vi "SL TAGS Open.vi"(8 "error in (no error)":errorcluster, 10 "Tag Properties":T1[](array[typedef]), 11 "EEISysLink in":refnum<class "EEISysLink.lvclass">) -> (0 "error out":errorcluster, 3 "EEISysLink out":refnum<class "EEISysLink.lvclass">)   [LabVIEW 2017, in "EEISysLink.lvclass"]
doc: "Open a local instance for each tag in a list per the input properties. Opened tags will be placed in the class data.\n\nThis does not synchronize them with a SystemLink server. To do that call the \"Ceate-Sync Server method\".\n\nJames Tillett\nEndeavor Engineering Inc.\nwww.endeavoreng.com"
uses:
  EEISysLink.lvclass
  Controls/SL Tag Properties.ctl
  Controls/SL Tag Data Type.ctl
  Controls/SL Tag Interpolation Method.ctl
  Controls/SL Tag Unit of Measure.ctl
  Controls/SL Tag Type.ctl
  <vilib>/Skyline/Configuration/Configuration_class/NI Skyline Configuration.lvclass
  <vilib>/Skyline/Configuration/Configuration AMQP_class/NI Skyline Configuration AMQP.lvclass
  C:/Program Files (x86)/National Instruments/LabVIEW 2017/vi.lib/Skyline/Configuration/Configuration_class/NI Skyline Configuration.lvclass
  <vilib>/Skyline/Configuration/Configuration AMQP_class/Open Configuration AMQP.vi
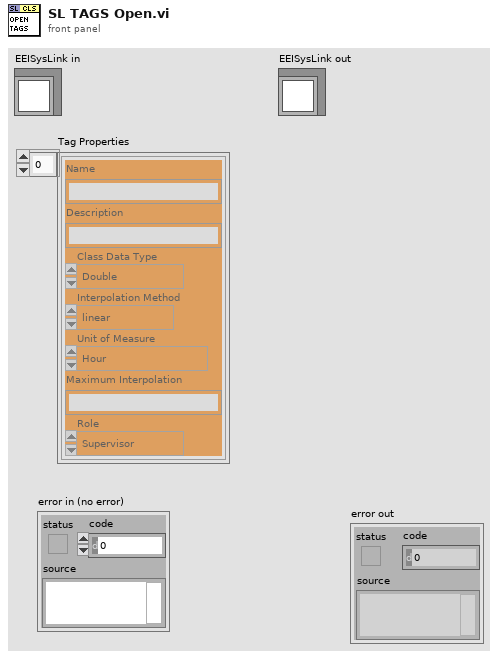
[diagram p1: front panel]
types:
  T1 = typedef "EEISysLink.lvclass/SL Tag Properties.ctl" = cluster{"Class Data Type":T2, "Name":string, "Description":string, "Interpolation Method":T3, "Unit of Measure":T4, "Maximum Interpolation":string, "Role":T5}
  T2 = typedef "EEISysLink.lvclass/SL Tag Data Type.ctl" = enum16{"Double", "Integer", "String", "Boolean", "Waveform"}
  T3 = typedef "EEISysLink.lvclass/SL Tag Interpolation Method.ctl" = enum16{"linear", "pilinear", "step"}
  T4 = typedef "EEISysLink.lvclass/SL Tag Unit of Measure.ctl" = enum16{"no units", "Second", "Hour", "Minute", "Day", "Year", "Month", "Week", "Foot", "Yard", "Meter", "Centimeter", "Inch", "Mile", "Nautical Mile", "Miles per Hour", "Meters per second", "Square meter", "Cubic meter", "Cubic centimeter", "Cubic inch", "Liter", "Gallon", "Gallons dry US", "Gallon UK", "Percent", "Revolutions per minute", "Revolution", "Degree angle", "Astronomical Unit", "Atom", "Atomic mass", "Bar", "Byte", "C (speed of light)", "Curie", "Decibel", "Electron Volt", "Ounce", "Knot", "G", "Grade", "Are", "Hectare", "Faraday", "Franklin", "Gilbert", "Erg", "Lambert", "Maxwell", "Gauss", "Electron mass", "Kilogram force", "Pound force", "Rad", "Centiradian", "Sphere", "Mach", "Fluid Ounces", "Fluid Ounces UK", "Fahrenheit", "Celsius", "Kelvin", "Rankine", "Gram", "Kilogram", "Pound", "Short/US Ton", "Long/UK ton", "Metric ton", "Mole", "Pounds per square inch", "Inches water column", "Torr", "Millitorr", "Millimeter mercury", "Inches mercury", "Bar (2)", "Atmosphere", "Pascal", "Watt", "kiloWatt", "Horsepower", "Kilowatt Hour", "British thermal units", "Millions of BTU", "Ampere", "Candela", "Radian", "Steradian", "Bit", "Hertz", "Newton", "Joule", "Coulomb", "Volt", "Farad", "Ohm", "Siemens", "Weber", "Tesla", "Henry", "Lumen", "Lux", "Becqueral", "Gray", "Sievert", "Katal", "Angstrom", "Light Year", "Parsec", "Point", "Pixel", "Dyne", "Kilogram force (2)", "Pound force (2)", "Rem", "Rutherford", "Roentgen"}
  T5 = typedef "EEISysLink.lvclass/SL Tag Type.ctl" = enum16{"All", "Supervisor", "Worker"}
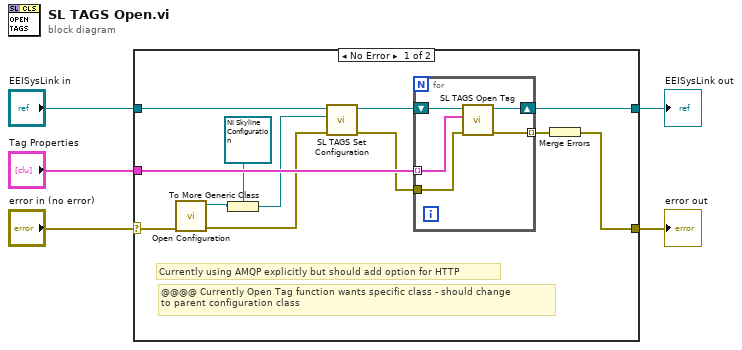
[diagram p0: block diagram]
diagram:
  n1 = case shown="No Error" "error in (no error)" {
    selector: "error in (no error)" -> [w11 w24]
    tunnel: [w15 w24] -> w4
    tunnel: [w14 w23] -> w2
    tunnel: "EEISysLink in" -> [w13 w23]
    tunnel: "Tag Properties" -> [w17 _]
    frame No Error {
      # "@@@@ Currently Open Tag function wants specific class - should change\nto parent configuration class"
      # "Currently using AMQP explicitly but should add option for HTTP"
      n2 = call-poly <vilib>:"Open Configuration.vi"("error in (no error)"=w11) -> ("error out"=w6:errorcluster, "AMQP configuration out"=w9:refnum<class "NI Skyline Configuration AMQP.lvclass">)  [unwired: 9 in]
      n3 = To More Generic Class(target class=refnum<class "NI Skyline Configuration.lvclass"> refnum ("Configuration"), reference=w9) -> (generic class reference=w7:refnum<class "NI Skyline Configuration.lvclass">)
      n4 = call-dynamic "SL TAGS Set Configuration.vi"("error in (no error)"=w6, "Configuration"=w7, "EEISysLink in"=w13) -> ("error out"=w10:errorcluster, "EEISysLink out"=w12:refnum<class "EEISysLink.lvclass">)  [unwired: 7 in]
      n5 = for {
        shift-right: [w19] -> w14
        shift-left: w12 -> [w22]
        tunnel: w17 -> [w21] mode=indexing
        tunnel: w10 -> [w20]
        tunnel: [w18] -> w16 mode=indexing
        n6 = call-dynamic "SL TAGS Open Tag.vi"("error in (no error)"=w20, "Tag Properties"=w21, "EEISysLink in"=w22) -> ("error out"=w18:errorcluster, "EEISysLink out"=w19:refnum<class "EEISysLink.lvclass">)  [unwired: 7 in]
      }
      n7 = Merge Errors(w16) -> (w15:errorcluster)
    }
    frame Error {
    }
  }
  "error out" <- w4
  "EEISysLink out" <- w2
